vi "Elevator Main.vi"   [LabVIEW 2013]
doc: "This is the main VI, it launches the modules that comprise the elevator application."
uses:
  Error Handler/Error_Control.ctl
  Database/DB_control.ctl
  Messaging/Msg_Control.ctl
types:
  T1 = typedef "Error_Control.ctl" = enum16{"Init", "Console_err", "Process_err", "Sensor_err"}
  T2 = typedef "Msg_Control.ctl" = enum16{"Init_Msg", "Sent_Inits", "Get_Ref", "Close_Ref"}
  T3 = typedef "DB_control.ctl" = enum16{"Initi_FGV", "Open", "Get_Data", "Write_Data", "Write_File", "Close_File"}
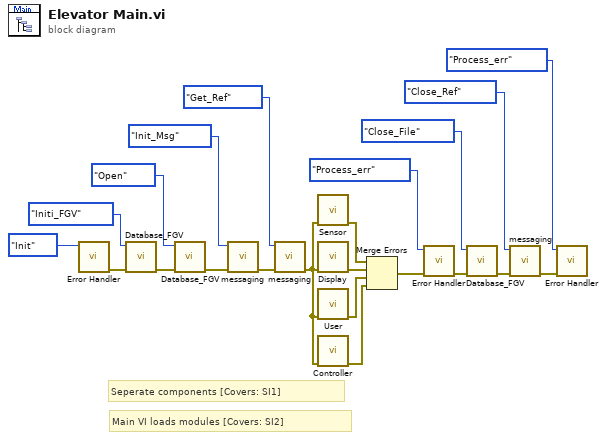
[diagram p0: block diagram]
diagram:
  # "Main VI loads modules [Covers: SI2]"
  # "Seperate components [Covers: SI1]"
  n1 = call "Error Handler.vi"("Error_Control"=Error_Control."Init") -> ("error out"=w21:errorcluster)  [unwired: 10 in]
  n2 = call "Database_FGV.vi"("error in (no error)"=w21, "DB Control"=DB_control."Initi_FGV") -> ("error out"=w15:errorcluster)  [unwired: 8 in, 1 out]
  n3 = call "Database_FGV.vi"("error in (no error)"=w15, "DB Control"=DB_control."Open") -> ("error out"=w14:errorcluster)  [unwired: 8 in, 1 out]
  n4 = call "messaging.vi"("error in (no error)"=w14, "Message_Control"=Msg_Control."Init_Msg") -> ("error out"=w18:errorcluster)  [unwired: 8 in, 1 out]
  n5 = call "messaging.vi"("error in (no error)"=w18, "Message_Control"=Msg_Control."Get_Ref") -> ("error out"=w13:errorcluster)  [unwired: 8 in, 1 out]
  n6 = call "Sensor.vi"("error in (no error)"=w13) -> ("error out"=w12:errorcluster)  [unwired: 10 in]
  n7 = call "Display.vi"("error in (no error)"=w13) -> ("error out"=w11:errorcluster)  [unwired: 10 in]
  n8 = call "User.vi"("error in (no error)"=w13) -> ("error out"=w10:errorcluster)  [unwired: 10 in]
  n9 = call "Controller.vi"("error in (no error)"=w13) -> ("error out"=w9:errorcluster)  [unwired: 10 in]
  n10 = Merge Errors(w12, w11, w10, w9) -> (w4:errorcluster)
  n11 = call "Error Handler.vi"("error in (no error)"=w4, "Error_Control"=Error_Control."Process_err") -> ("error out"=w3:errorcluster)  [unwired: 9 in]
  n12 = call "Database_FGV.vi"("error in (no error)"=w3, "DB Control"=DB_control."Close_File") -> ("error out"=w7:errorcluster)  [unwired: 8 in, 1 out]
  n13 = call "messaging.vi"("error in (no error)"=w7, "Message_Control"=Msg_Control."Close_Ref") -> ("error out"=w2:errorcluster)  [unwired: 8 in, 1 out]
  n14 = call "Error Handler.vi"("error in (no error)"=w2, "Error_Control"=Error_Control."Process_err") -> ()  [unwired: 9 in, 1 out]
